vi "Test Target has two Missmatching Sections.vi"(11 "Test Case In":refnum<class "Added Section Finder Test.lvclass">) -> (0 "error out":errorcluster, 3 "Test Case Out":refnum<class "Added Section Finder Test.lvclass">)   [LabVIEW 2020, in "Added Section Finder Test.lvclass"]
uses:
  Added Section Finder Test.lvclass
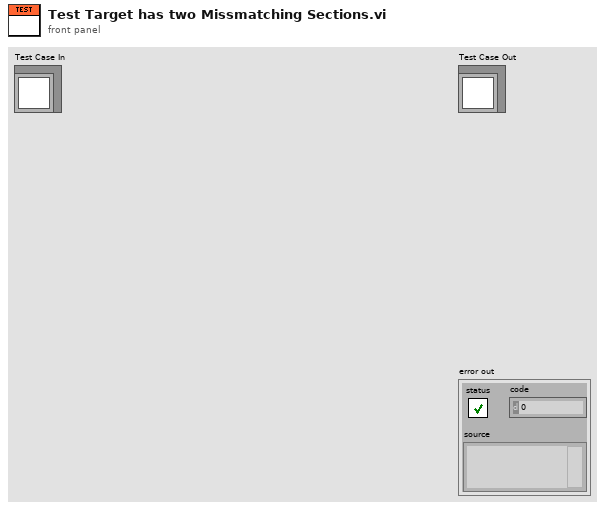
[diagram p1: front panel]
types:
  T1 = cluster{"Selection Start":u32, "Selection End":u32}
  T2 = cluster{"Selection Start":u32, "Selection End":u32}[]
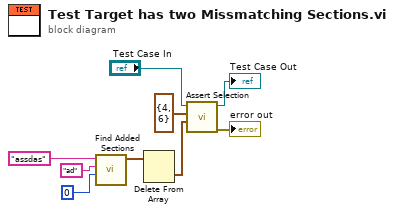
[diagram p0: block diagram]
diagram:
  n1 = call "Find Added Sections.vi"("Offset"=u32 0 ("Index"), "Reference"="ad", "Target"="assdas") -> ("Sections in Target"=w8:T2)  [unwired: 8 in]
  n2 = Delete From Array(array=w8) -> (deleted portion=w3:T1)  [unwired: 2 in, 1 out]
  n3 = call "Assert Selection.vi"("Actual"=w3, "Expected"=T1 {"Selection Start"=4, "Selection End"=6} ("Text.Selection"), "Added Section Finder Test In"="Test Case In") -> ("error out"=→"error out":errorcluster, "Added Section Finder Test Out"=→"Test Case Out":refnum<class "Added Section Finder Test.lvclass">)  [unwired: 7 in]
